vi "Create State and Input String Maps.vi"(8 "error in (no error)":errorcluster, 9 "Input Strings":string[](array[string]), 10 "State Strings":string[](array[string]), 11 "StateMachine in":refnum<class "StateMachine.lvclass">) -> (0 "error out":errorcluster, 3 "StateMachine out":refnum<class "StateMachine.lvclass">)   [LabVIEW 2019, in "State Machine.lvlib" / "StateMachine.lvclass"]
uses:
  StateMachine.lvclass
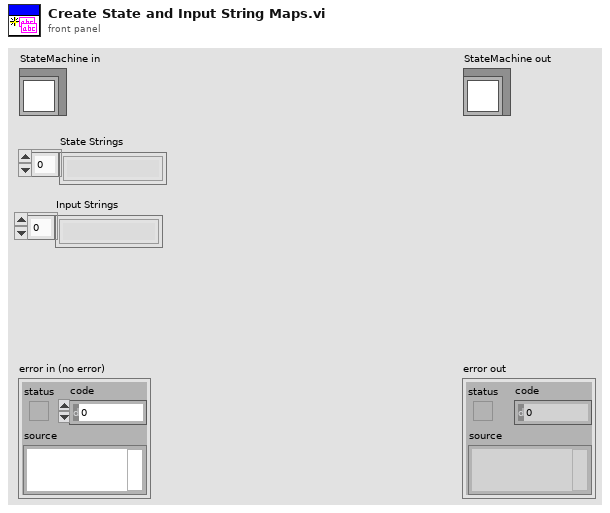
[diagram p1: front panel]
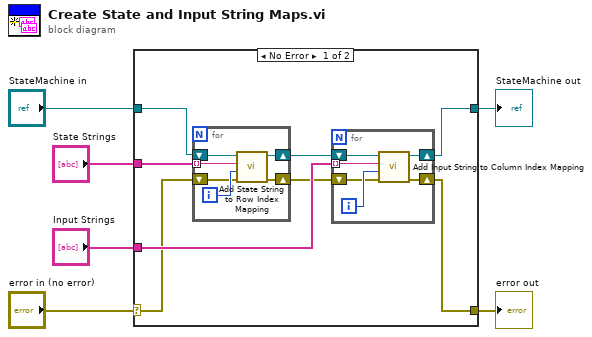
[diagram p0: block diagram]
diagram:
  n1 = case shown="No Error" "error in (no error)" {
    selector: "error in (no error)" -> [w10 w28]
    tunnel: [w8 w28] -> w5
    tunnel: [w7 w27] -> w3
    tunnel: "StateMachine in" -> [w13 w27]
    tunnel: "State Strings" -> [w14 _]
    tunnel: "Input Strings" -> [w12 _]
    frame No Error {
      n2 = for {
        tunnel: w14 -> [w19] mode=indexing
        shift-right: [w17] -> w11
        shift-left: w13 -> [w18]
        shift-right: [w15] -> w9
        shift-left: w10 -> [w16]
        i -> [w20]
        n3 = call-dynamic "Add State String to Row Index Mapping.vi"("error in (no error)"=w16, "Row Index"=w20, "State String"=w19, "StateMachine in"=w18) -> ("error out"=w15:errorcluster, "StateMachine out"=w17:refnum<class "StateMachine.lvclass">)  [unwired: 5 in, 1 out]
      }
      n4 = for {
        tunnel: w12 -> [w26] mode=indexing
        shift-right: [w22] -> w7
        shift-left: w11 -> [w25]
        shift-right: [w21] -> w8
        shift-left: w9 -> [w23]
        i -> [w24]
        n5 = call-dynamic "Add Input String to Column Index Mapping.vi"("error in (no error)"=w23, "Row Index"=w24, "State String"=w26, "StateMachine in"=w25) -> ("error out"=w21:errorcluster, "StateMachine out"=w22:refnum<class "StateMachine.lvclass">)  [unwired: 5 in, 1 out]
      }
    }
    frame Error {
    }
  }
  "error out" <- w5
  "StateMachine out" <- w3
